vi "PM100D_Plot_ph.vi"(1 "Beam Name":string="Green Unshifted") -> ()   [LabVIEW 2010]
doc: "This VI shows how to communicate with a PM100D optical power/energy meter with SCPI commands.\n- Initializing the instrument\n- Getting system info\n- Setting parameters\n- Measurement configuration\n- Measuring queue\n- Fetching and displaying a measurement value\n- Closing the application"
panel:
  in  "Publish As Adam Channel":bool
  out "Wavelength nm":string="488"
  out "Waveform Chart":dbl(graph)
  out "Readout value":dbl format="%^#_9e"
  out "IDN String":string
  out "Sensor SN":string
  out "Sensor Name":string
  out "Sensor Flags":bool[](array[boolean])
  out "New":bool
  in  "Timeout [ms]":i32=1000
  in  "stop":bool
  in  "Readout Config":string(combo)="POW"
  out "Readout string":string
  out "Error log":string
  in  "Averaging Rate":i32=300
  # "1 Power Sensor"
  # "2 Energy Sensor"
  # "4"
  # "8"
  # "16 Response settable"
  # "32 Wavelength settable"
  # "64 Tau (time constant) settable"
  # "128"
  # "256 With temperature sensor"
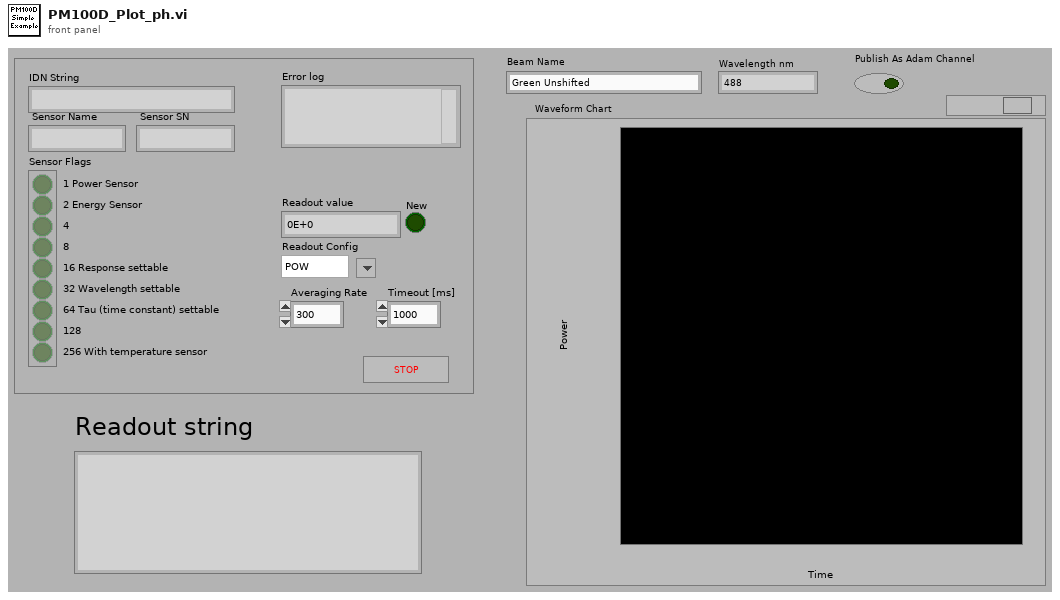
[diagram p1: front panel]
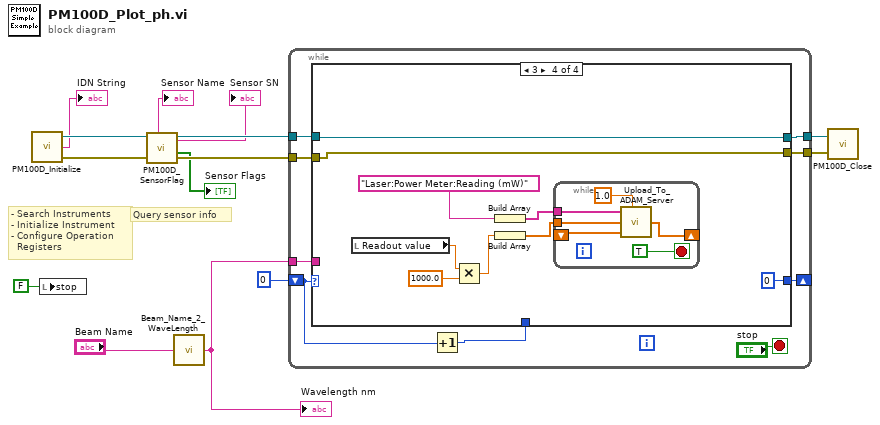
[diagram p0: block diagram]
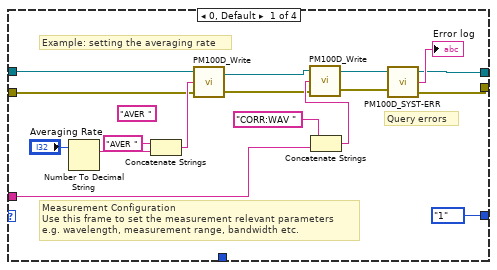
[diagram p2: hidden frame]
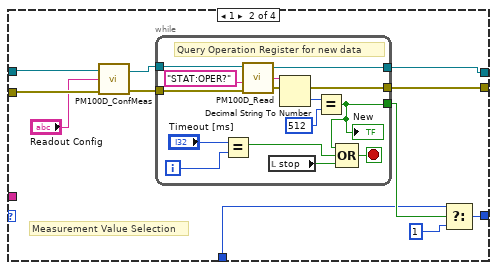
[diagram p3: hidden frame]
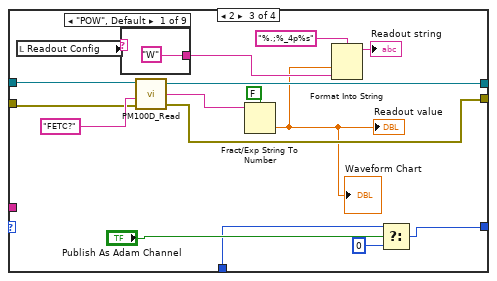
[diagram p4: hidden frame]
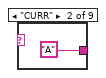
[diagram p5: hidden frame]
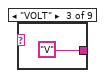
[diagram p6: hidden frame]
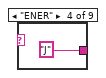
[diagram p7: hidden frame]
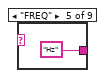
[diagram p8: hidden frame]
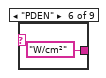
[diagram p9: hidden frame]
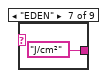
[diagram p10: hidden frame]
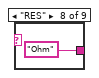
[diagram p11: hidden frame]
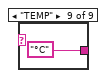
[diagram p12: hidden frame]
diagram:
  # "- Search Instruments\n- Initialize Instrument\n- Configure Operation\n  Registers"
  # "Query sensor info"
  n1 = call "PM100D_Initialize.vi"() -> ("error out"=w13:errorcluster, "Instrument"=→"IDN String":string, "VISA out"=w14:refnum<visa-resource-name>)  [unwired: 3 out]
  n2 = local write "stop"(FALSE ("stop")) -> ()
  n3 = call "PM100D_SensorFlag.vi"("error in (no error)"=w13, "VISA in"=w14) -> ("error out"=w11:errorcluster, "flags"=→"Sensor Flags":bool[], "VISA out"=w12:refnum<visa-resource-name>, "sn"=→"Sensor SN":string, "name"=→"Sensor Name":string)  [unwired: 5 out]
  n4 = call "Beam_Name_2_WaveLength.vi"("Beam Name"="Beam Name") -> ("Wavelength nm"=w2:string)
  "Wavelength nm" <- w2
  n5 = while {
    tunnel: w12 -> [w23]
    tunnel: w11 -> [w22]
    shift-right: [w20] -> _
    shift-left: 0 -> [w16]
    tunnel: [w19] -> w6
    tunnel: [w18] -> w5
    tunnel: w2 -> [w17]
    stop <- "stop" stop-if-true
    n6 = Increment(x=w16) -> (x+1=w15:i32)
    n7 = case shown="3" w16 {
      tunnel: w23 -> [w37 w51 w80 w99]
      tunnel: w22 -> [w34 w50 w79 w98]
      tunnel: [enum16{"0", "1", "2"}."1" w45 w68 0 ("f")] -> w20
      tunnel: [w32 w47 w78 w99] -> w19
      tunnel: [w31 w46 w71 w98] -> w18
      tunnel: w17 -> [w28 _ _ _]
      tunnel: w15 -> [_ w42 w67 _]
      frame 0, Default {
        (unwired) "AVER " ("string")
        # "Query errors"
        # "Example: setting the averaging rate"
        # "Measurement Configuration\nUse this frame to set the measurement relevant parameters\ne.g. wavelength, measurement range, bandwidth etc."
        n8 = Number To Decimal String(number="Averaging Rate") -> (decimal integer string=w39:string)  [unwired: 1 out]
        n9 = Concatenate Strings("AVER " ("string"), w39) -> (w36:string)
        n10 = call "PM100D_Write.vi"("error in (no error)"=w34, "Command"=w36, "VISA in"=w37) -> ("error out"=w26:errorcluster, "VISA out"=w27:refnum<visa-resource-name>)
        n11 = Concatenate Strings("CORR:WAV " ("string"), w28) -> (w30:string)
        n12 = call "PM100D_Write.vi"("error in (no error)"=w26, "Command"=w30, "VISA in"=w27) -> ("error out"=w25:errorcluster, "VISA out"=w24:refnum<visa-resource-name>)
        n13 = call "PM100D_SYST-ERR.vi"("error out 2"=w25, "VISA In"=w24) -> ("error out"=w31:errorcluster, "Error"=→"Error log":string, "VISA Out"=w32:refnum<visa-resource-name>)  [unwired: 1 out]
      }
      frame 1 {
        # "Measurement Value Selection"
        n14 = call "PM100D_ConfMeas.vi"("error in"=w50, "Conf:"="Readout Config", "VISA In"=w51) -> ("error out"=w48:errorcluster, "dup VISA session"=w49:refnum<visa-resource-name>)
        n15 = while {
          tunnel: w49 -> [w61]
          tunnel: w48 -> [w60]
          tunnel: [w59] -> w47
          tunnel: [w58] -> w46
          tunnel: [w52] -> w44
          i -> [w54]
          stop <- w56 stop-if-true
          # "Query Operation Register for new data"
          n16 = Equal?(x="Timeout [ms]", y=w54) -> (x = y?=w53:bool)
          n17 = call "PM100D_Read.vi"("error in (no error)"=w60, "Command"="STAT:OPER?", "VISA in"=w61) -> ("error out"=w58:errorcluster, "ReadValue"=w64:string, "VISA out"=w59:refnum<visa-resource-name>)  [unwired: 1 out]
          n18 = local read "stop"() -> (w57:bool)
          n19 = Decimal String To Number(string=w64) -> (number=w63:i32)  [unwired: 1 in, 2 out]
          n20 = Equal?(x=w63, y=512) -> (x = y?=w52:bool)
          "New" <- w52
          n21 = Compound Arithmetic op=OR(w52, w53, w57) -> (w56:bool)
        }
        n22 = Select(t=w42, s=w44, f=1) -> (s? t:f=w45:i32)
      }
      frame 2 {
        n23 = local read "Readout Config"() -> (w77:string)
        n24 = case shown="\"POW\", Default" w77 {
          tunnel: ["W" "A" "V" "J" "Hz" "W/cm²" "J/cm²" "Ohm" "°C"] -> w73
          frame "POW", Default {
          }
          frame "CURR" {
          }
          frame "VOLT" {
          }
          frame "ENER" {
          }
          frame "FREQ" {
          }
          frame "PDEN" {
          }
          frame "EDEN" {
          }
          frame "RES" {
          }
          frame "TEMP" {
          }
        }
        n25 = call "PM100D_Read.vi"("error in (no error)"=w79, "Command"="FETC?", "VISA in"=w80) -> ("error out"=w71:errorcluster, "ReadValue"=w76:string, "VISA out"=w78:refnum<visa-resource-name>)  [unwired: 1 out]
        n26 = Fract/Exp String To Number(use system decimal point (T)=FALSE, string=w76) -> (number=w70:dbl)  [unwired: 3 out]
        "Readout value" <- w70
        "Waveform Chart" <- w70
        n27 = Format Into String(format string="%.;%_4p%s", w70, w73) -> (resulting string=→"Readout string":string)  [unwired: 2 in, 1 out]
        n28 = Select(t=w67, s="Publish As Adam Channel", f=0) -> (s? t:f=w68:i32)
      }
      frame 3 {
        n29 = local read "Readout value"() -> (w93:dbl)
        n30 = Multiply(x=w93, y=1000.0) -> (x*y=w91:dbl)
        n31 = Build Array("Laser:Power Meter:Reading (mW)" ("String")) -> (w94:string[])
        n32 = Build Array(w91) -> (w95:dbl[])
        n33 = while {
          shift-right: [w105] -> _
          shift-left: _ -> [w104]
          tunnel: w95 -> [w101]
          tunnel: w94 -> [w100]
          stop <- TRUE stop-if-true
          n34 = call "Upload_To_ADAM_Server.vi"("Channel Names"=w100, "Averaging Period (s)"=1.0, "Channel Values"=w101, "Shift In"=w104) -> ("Shift Out"=w105:dbl[])  [unwired: 1 out]
        }
      }
    }
  }
  n35 = call "PM100D_Close.vi"("error in (no error)"=w5, "VISA resource name"=w6) -> ()  [unwired: 1 in, 1 out]
